vi "Main.vi"() -> ()   [LabVIEW 2017]
uses:
  Access Factory/Access Factory.lvclass
  SQL Factory/SQL Factory.lvclass
  Abstract Department/Abstract Department.lvclass
  Abstract User/Abstract User.lvclass
panel:
  in  "SQL InsertDp":bool
  in  "SQL GetDp":bool
  in  "Access InsertDp":bool
  in  "Access GetDp":bool
  in  "SQL InsertUser":bool
  in  "SQL GetUser":bool
  in  "Access InsertUser":bool
  in  "Access GetUser":bool
  out "字符串":string
  # "User表"
  # "Access"
  # "SQL"
  # "Department表"
  # "Access"
  # "SQL"
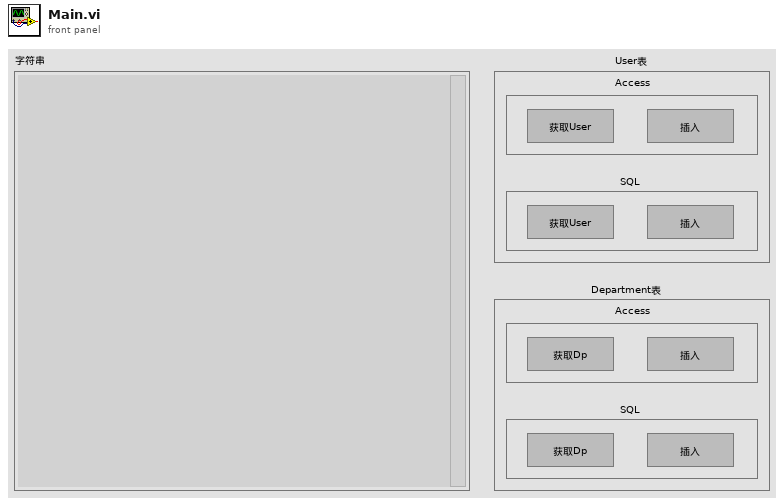
[diagram p1: front panel]
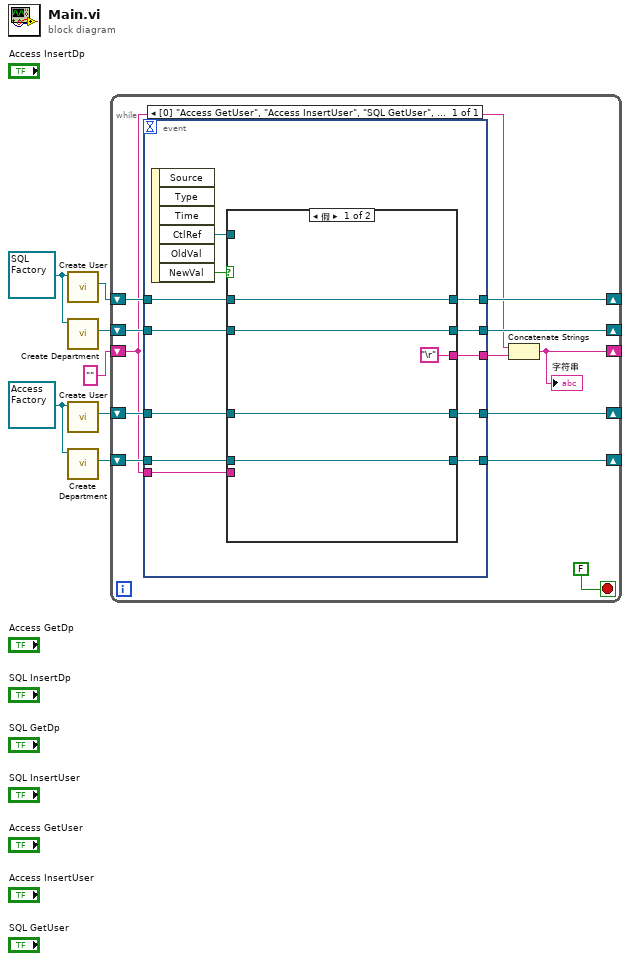
[diagram p0: block diagram]
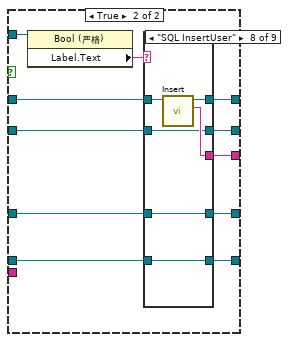
[diagram p2: hidden frame]
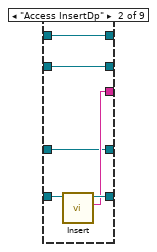
[diagram p4: hidden frame]
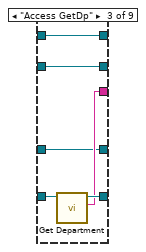
[diagram p5: hidden frame]
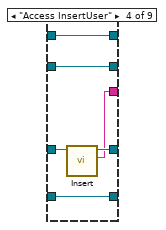
[diagram p6: hidden frame]
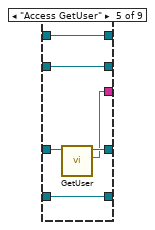
[diagram p7: hidden frame]
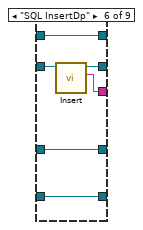
[diagram p8: hidden frame]
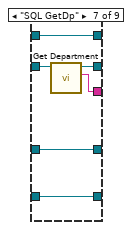
[diagram p9: hidden frame]
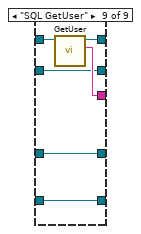
[diagram p10: hidden frame]
diagram:
  w3 = refnum<class "SQL Factory.lvclass"> refnum ("SQL Factory.lvclass")
  w5 = refnum<class "Access Factory.lvclass"> refnum ("Access Factory.lvclass")
  n1 = call-dynamic "Create User.vi"("SQL Factory 输入"=w3) -> ("Abstract User.lvclass"=w1:refnum<class "Abstract User.lvclass">)  [unwired: 8 in, 2 out]
  n2 = call-dynamic "Create Department.vi"("SQL Factory 输入"=w3) -> ("Abstract Department.lvclass"=w2:refnum<class "Abstract Department.lvclass">)  [unwired: 8 in, 2 out]
  n3 = call-dynamic "Create User.vi"("Access Factory 输入"=w5) -> ("Abstract User.lvclass"=w4:refnum<class "Abstract User.lvclass">)  [unwired: 8 in, 2 out]
  n4 = call-dynamic "Create Department.vi"("Access Factory 输入"=w5) -> ("Abstract Department.lvclass"=w6:refnum<class "Abstract Department.lvclass">)  [unwired: 8 in, 2 out]
  n5 = while {
    shift-right: [w10] -> _
    shift-left: "" -> [w8]
    shift-right: [w17] -> _
    shift-left: w2 -> [w13]
    shift-right: [w18] -> _
    shift-left: w6 -> [w11]
    shift-right: [w19] -> _
    shift-left: w4 -> [w12]
    shift-right: [w16] -> _
    shift-left: w1 -> [w14]
    stop <- FALSE stop-if-true
    n6 = event shown="[0] \"Access GetUser\", \"Access InsertUser\", \"SQL GetUser\", \"SQL InsertUser\", \"Access GetDp\", \"Access InsertDp\", \"SQL InsertDp\", \"SQL GetDp\": 值改变" {
      selector: _ -> [_]
      dyn-events: _ -> [_]
      timeout: _ -> [_]
      tunnel: w11 -> [w30]
      tunnel: w12 -> [w29]
      tunnel: [w28] -> w19
      tunnel: [w27] -> w18
      tunnel: [w26] -> w9
      tunnel: [w25] -> w17
      tunnel: w14 -> [w24]
      tunnel: [w23] -> w16
      tunnel: w13 -> [w22]
      tunnel: w8 -> [w20]
      event "Access GetUser", "Access InsertUser", "SQL GetUser", "SQL InsertUser", "Access GetDp", "Access InsertDp", "SQL InsertDp", "SQL GetDp": Value Change {
        n7 = event-data() -> ("CtlRef"=w31:refnum<vi>, "NewVal"=w21:bool)  [unwired: 1 in, 4 out]
        n8 = case shown="假" w21 {
          tunnel: w31 -> [_ w47]
          tunnel: w30 -> [w33 w45]
          tunnel: w29 -> [w34 w44]
          tunnel: [w34 w43] -> w28
          tunnel: [w33 w42] -> w27
          tunnel: ["\r" w41] -> w26
          tunnel: [w35 w40] -> w25
          tunnel: w24 -> [w36 w39]
          tunnel: [w36 w38] -> w23
          tunnel: w22 -> [w35 w37]
          tunnel: w20 -> [_ _]
          frame False {
          }
          frame True {
            n9 = property class="Bool (严格)"(reference=w47) -> ("Label.Text"=w46:string)  [unwired: 1 in, 2 out]
            n10 = case shown="\"SQL InsertUser\"" w46 {
              tunnel: w45 -> [w50 w57 w63 w64 w70 w76 w82 w88 w94]
              tunnel: w44 -> [w51 w52 w58 w69 w75 w77 w83 w89 w95]
              tunnel: [w51 w52 w58 w68 w74 w77 w83 w89 w95] -> w43
              tunnel: [w50 w56 w62 w64 w70 w76 w82 w88 w94] -> w42
              tunnel: [_ w55 w61 w67 w73 w80 w86 w92 w98] -> w41
              tunnel: w37 -> [w49 w53 w59 w65 w71 w81 w87 w90 w96]
              tunnel: [w49 w53 w59 w65 w71 w79 w85 w90 w96] -> w40
              tunnel: w39 -> [w48 w54 w60 w66 w72 w78 w84 w93 w99]
              tunnel: [w48 w54 w60 w66 w72 w78 w84 w91 w97] -> w38
              frame Default {
              }
              frame "Access InsertDp" {
                n11 = call-dynamic "Insert.vi"("Abstract Department 输入"=w57) -> ("字符串"=w55:string, "Abstract Department 输出"=w56:refnum<class "Abstract Department.lvclass">)  [unwired: 8 in, 1 out]
              }
              frame "Access GetDp" {
                n12 = call-dynamic "Get Department.vi"("Abstract Department 输入"=w63) -> ("字符串"=w61:string, "Abstract Department 输出"=w62:refnum<class "Abstract Department.lvclass">)  [unwired: 8 in, 1 out]
              }
              frame "Access InsertUser" {
                n13 = call-dynamic "Insert.vi"("Abstract User 输入"=w69) -> ("字符串"=w67:string, "Abstract User 输出"=w68:refnum<class "Abstract User.lvclass">)  [unwired: 8 in, 1 out]
              }
              frame "Access GetUser" {
                n14 = call-dynamic "GetUser.vi"("Abstract User 输入"=w75) -> ("字符串"=w73:string, "Abstract User 输出"=w74:refnum<class "Abstract User.lvclass">)  [unwired: 8 in, 1 out]
              }
              frame "SQL InsertDp" {
                n15 = call-dynamic "Insert.vi"("Abstract Department 输入"=w81) -> ("字符串"=w80:string, "Abstract Department 输出"=w79:refnum<class "Abstract Department.lvclass">)  [unwired: 8 in, 1 out]
              }
              frame "SQL GetDp" {
                n16 = call-dynamic "Get Department.vi"("Abstract Department 输入"=w87) -> ("字符串"=w86:string, "Abstract Department 输出"=w85:refnum<class "Abstract Department.lvclass">)  [unwired: 8 in, 1 out]
              }
              frame "SQL InsertUser" {
                n17 = call-dynamic "Insert.vi"("Abstract User 输入"=w93) -> ("字符串"=w92:string, "Abstract User 输出"=w91:refnum<class "Abstract User.lvclass">)  [unwired: 8 in, 1 out]
              }
              frame "SQL GetUser" {
                n18 = call-dynamic "GetUser.vi"("Abstract User 输入"=w99) -> ("字符串"=w98:string, "Abstract User 输出"=w97:refnum<class "Abstract User.lvclass">)  [unwired: 8 in, 1 out]
              }
            }
          }
        }
      }
    }
    n19 = Concatenate Strings(w8, w9) -> (w10:string)
    "字符串" <- w10
  }
